vi "SMS Image Preview Select ROI.vi"(7 "Camera Image Ref":T2) -> (4 "Camera ROI":T1, 15 "Canceled?":bool)   [LabVIEW 2020]
uses:
  <vilib>/vision/Image Controls.llb/IMAQ Image.ctl
  <vilib>/Utility/miscctls.llb/LVPointTypeDef.ctl
panel:
  in  "Tool Selection":enum32{"Zoom Tool", "ROI Tool", "Pan Tool"}(radio)
  in  "Cancel":bool
  in  "Done":bool
  out "Camera Display":T2(plugin-control)
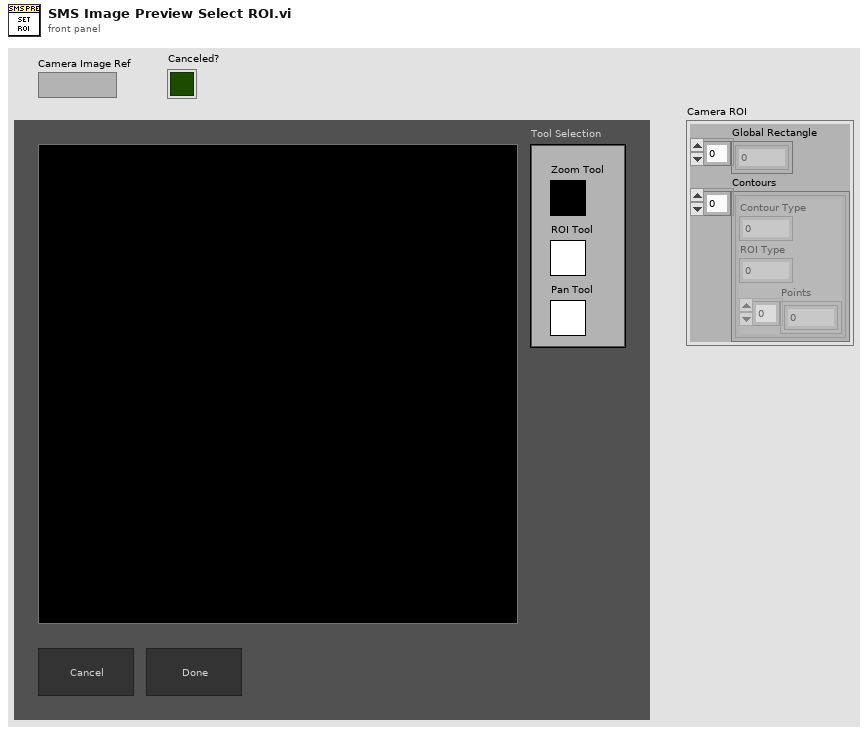
[diagram p1: front panel]
types:
  T1 = cluster{"Global Rectangle":i32[], "Contours":cluster{"Contour Type":u32, "ROI Type":u32, "Points":i32[]}[]}
  T2 = typedef "IMAQ Image.ctl" = refnum<image>
  T3 = enum16{"Always On", "Always Off", "Off While Running"}
  T4 = typedef "LVPointTypeDef.ctl" = cluster{"Horizontal":i16, "Vertical":i16}
  T5 = typedef "LVRectTypeDef.ctl" = cluster{"Left":i16, "Top":i16, "Right":i16, "Bottom":i16}
  T6 = typedef "LVBoundsTypeDef.ctl" = cluster{"Width":u32, "Height":u32}
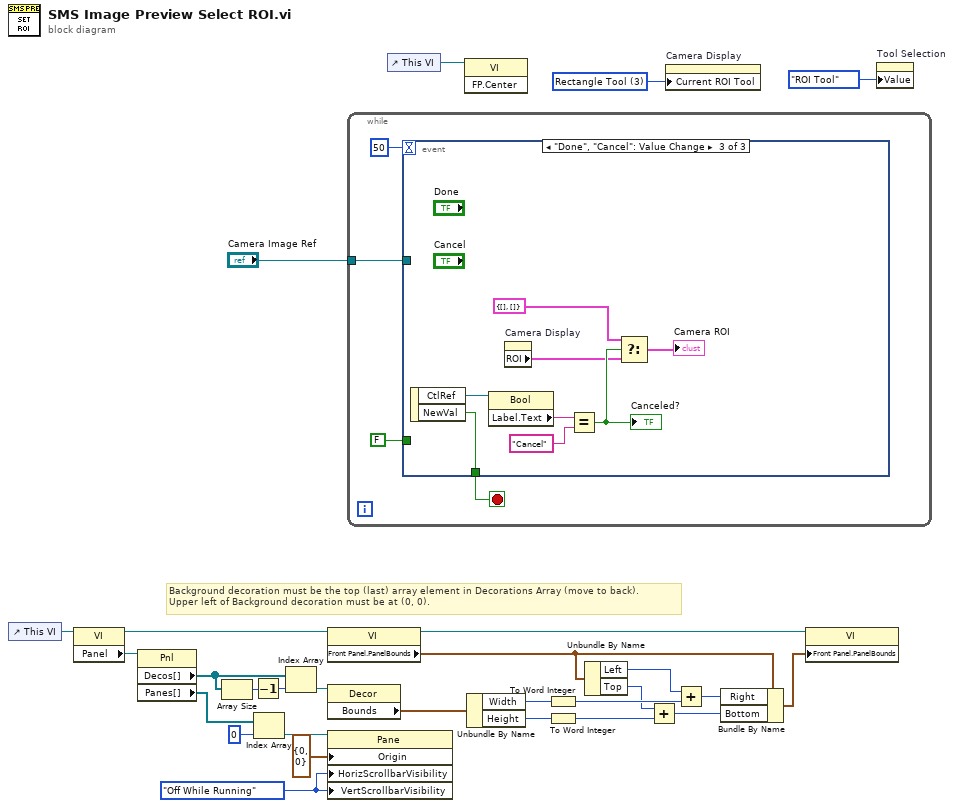
[diagram p0: block diagram]
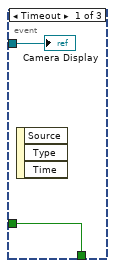
[diagram p2: hidden frame]
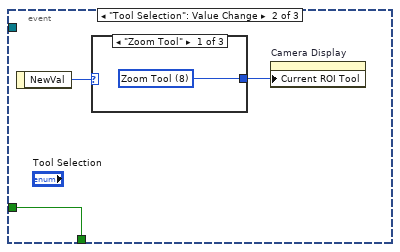
[diagram p3: hidden frame]
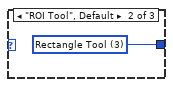
[diagram p4: hidden frame]
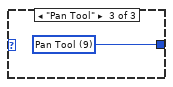
[diagram p5: hidden frame]
diagram:
  w14 = T3."Off While Running" ("Vertical Scrollbar Visibility")
  w28 = u32 3 items=["Zoom Tool"=8, "Selection Tool"=0, "Pan Tool"=9, "Point Tool"=1, "Line Tool"=2, "Rectangle Tool"=3, "Rotated Rectangle Tool"=12, "Polyline Tool"=10, "Polygon Tool"=5, "Freehand Tool"=11, "Closed Freehand Tool"=6, "Ellipse Tool"=4, "Annulus Tool"=7] ("Current ROI Tool")
  # "Background decoration must be the top (last) array element in Decorations Array (move to back).\nUpper left of Background decoration must be at (0, 0)."
  n1 = control-ref of="This VI"() -> (w7:refnum<vi>)
  n2 = property class="VI"(reference=w7) -> (reference out=w15:refnum<vi>, "Panel"=w8:refnum<vi>)  [unwired: 1 in, 1 out]
  n3 = property class="Pnl"(reference=w8) -> ("Decos[]"=w6:refnum<vi>[], "Panes[]"=w11:refnum<vi>[])  [unwired: 1 in, 2 out]
  n4 = Array Size(array=w6) -> (size(s)=w4:i32)
  n5 = Decrement(x=w4) -> (x-1=w5:i32)
  n6 = Index Array(array=w11, index=0) -> (element=w10:refnum<vi>)
  n7 = Index Array(array=w6, index=w5) -> (element=w13:refnum<vi>)
  n8 = property class="VI"(reference=w15) -> (reference out=w17:refnum<vi>, "Front Panel.PanelBounds"=w18:T5)  [unwired: 1 in, 1 out]
  n9 = property class="Decor"(reference=w13) -> ("Bounds"=w16:T6)  [unwired: 1 in, 2 out]
  n10 = property class="Pane"(reference=w10, "Origin"=T4 {"Horizontal"=0, "Vertical"=0}, "HorizScrollbarVisibility"=w14, "VertScrollbarVisibility"=w14) -> ()  [unwired: 1 in, 2 out]
  n11 = while {
    tunnel: "Camera Image Ref" -> [w30]
    stop <- w32 stop-if-true
    n12 = event shown="[2] \"Done\", \"Cancel\": Value Change" {
      selector: _ -> [_ _ _]
      dyn-events: _ -> [_ _ _]
      timeout: 50 -> [_ _ _]
      tunnel: [w34 w37 w45] -> w32
      tunnel: FALSE -> [w34 w37 _]
      tunnel: w30 -> [w33 _ _]
      event Timeout {
        n13 = event-data() -> ()  [unwired: 1 in, 3 out]
        "Camera Display" <- w33
      }
      event "Tool Selection": Value Change {
        n14 = event-data() -> ("NewVal"=w36:enum32{"Zoom Tool", "ROI Tool", "Pan Tool"})  [unwired: 1 in]
        n15 = case shown="\"Zoom Tool\"" w36 {
          tunnel: [w38 w39 w40] -> w35
          frame "Zoom Tool" {
            w38 = u32 8 items=["Zoom Tool"=8, "Selection Tool"=0, "Pan Tool"=9, "Point Tool"=1, "Line Tool"=2, "Rectangle Tool"=3, "Rotated Rectangle Tool"=12, "Polyline Tool"=10, "Polygon Tool"=5, "Freehand Tool"=11, "Closed Freehand Tool"=6, "Ellipse Tool"=4, "Annulus Tool"=7] ("Current ROI Tool")
          }
          frame "ROI Tool", Default {
            w39 = u32 3 items=["Zoom Tool"=8, "Selection Tool"=0, "Pan Tool"=9, "Point Tool"=1, "Line Tool"=2, "Rectangle Tool"=3, "Rotated Rectangle Tool"=12, "Polyline Tool"=10, "Polygon Tool"=5, "Freehand Tool"=11, "Closed Freehand Tool"=6, "Ellipse Tool"=4, "Annulus Tool"=7] ("Current ROI Tool")
          }
          frame "Pan Tool" {
            w40 = u32 9 items=["Zoom Tool"=8, "Selection Tool"=0, "Pan Tool"=9, "Point Tool"=1, "Line Tool"=2, "Rectangle Tool"=3, "Rotated Rectangle Tool"=12, "Polyline Tool"=10, "Polygon Tool"=5, "Freehand Tool"=11, "Closed Freehand Tool"=6, "Ellipse Tool"=4, "Annulus Tool"=7] ("Current ROI Tool")
          }
        }
        n16 = property on="Camera Display" class="ImageControl"("Current ROI Tool"=w35) -> ()  [unwired: 2 in, 2 out]
      }
      event "Done", "Cancel": Value Change {
        n17 = event-data() -> ("CtlRef"=w48:refnum<vi>, "NewVal"=w45:bool)  [unwired: 1 in]
        n18 = property class="Bool"(reference=w48) -> ("Label.Text"=w47:string)  [unwired: 1 in, 2 out]
        n19 = property on="Camera Display" class="ImageControl"() -> ("ROI"=w43:T1)  [unwired: 2 in, 2 out]
        n20 = Equal?(x=w47, y="Cancel") -> (x = y?=w44:bool)
        "Canceled?" <- w44
        n21 = Select(t=T1 {"Global Rectangle"=[], "Contours"=[]} ("Camera ROI"), s=w44, f=w43) -> (s? t:f=→"Camera ROI":T1)
      }
    }
  }
  n22 = control-ref of="This VI"() -> (w26:refnum<vi>)
  n23 = invoke class="VI" method="FP.Center"(reference=w26) -> ()  [unwired: 2 in, 3 out]
  n24 = Unbundle By Name(w16) -> ("Width"=w21:u32, "Height"=w24:u32)
  n25 = To Word Integer(number=w21) -> (16bit integer=w23:i16)
  n26 = To Word Integer(number=w24) -> (16bit integer=w1:i16)
  n27 = Unbundle By Name(w18) -> ("Left"=w20:i16, "Top"=w3:i16)
  n28 = Add(x=w3, y=w1) -> (x+y=w2:i16)
  n29 = property on="Camera Display" class="ImageControl"("Current ROI Tool"=w28) -> ()  [unwired: 2 in, 2 out]
  n30 = Add(x=w20, y=w23) -> (x+y=w22:i16)
  n31 = Bundle By Name(cluster=w18, "Right"=w22, "Bottom"=w2) -> (w19:T5)
  n32 = property class="VI"(reference=w17, "Front Panel.PanelBounds"=w19) -> ()  [unwired: 1 in, 2 out]
  n33 = property on="Tool Selection" class="RadioBtnsControl (strict)"("Value"=enum32{"Zoom Tool", "ROI Tool", "Pan Tool"}."ROI Tool" ("Tool Selection")) -> ()  [unwired: 2 in, 2 out]
